vi "Trigger Broadcast.vi"(8 "error in (no error)":errorcluster, 11 "Process in":refnum<class "Debug Process.lvclass">) -> (0 "error out":errorcluster, 3 "Process out":refnum<class "Debug Process.lvclass">)   [LabVIEW 2020, in "Debug Process.lvclass"]
doc: "Execute the Trigger Broadcast Event state of the process. This may be used for updating the current status or state of the process to all subscribed observers."
uses:
  Debug Process.lvclass
  Debug Process.lvclass/Debug Process.ctl
  Lifecycle/Get Lifecycle State.vi
  <vilib>/Utility/error.llb/Clear Errors.vi
  <vilib>/Utility/error.llb/Error Cluster From Error Code.vi
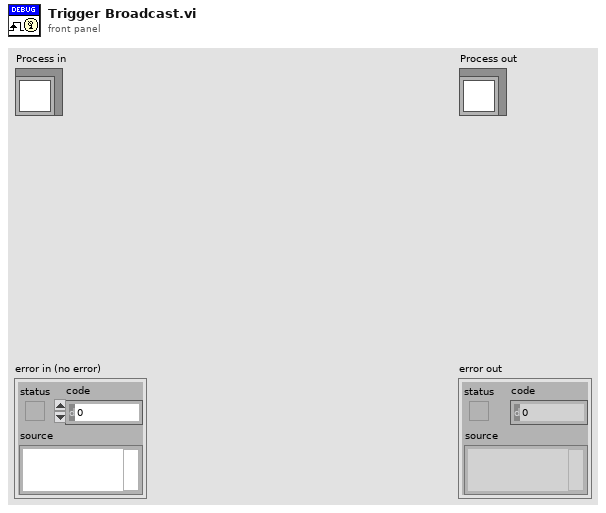
[diagram p1: front panel]
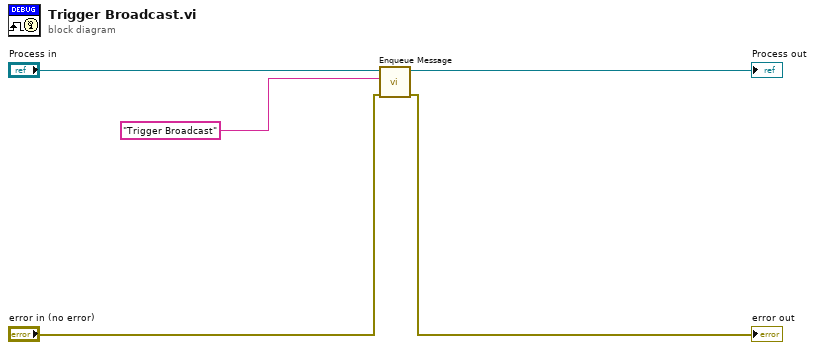
[diagram p0: block diagram]
diagram:
  n1 = call "Enqueue Message.vi"("error in (no error)"="error in (no error)", "Message"="Trigger Broadcast", "Process In"="Process in") -> ("error out"=→"error out":errorcluster, "Process Out"=→"Process out":refnum<class "Debug Process.lvclass">)  [unwired: 7 in]
